vi "Get Channels from Line.vi"(11 "Line":T1={"channel"=refnum, "XNET Signal"="CANEventSignal1\nNIXNET_example.CAN_Cluster"}) -> (3 "Channels":refnum<class "TBM channel.lvclass">[](array[class]))   [LabVIEW 2014, in "J1939 configuration.lvclass"]
doc: "Returns an array of channels for a single line."
uses:
  J1939 configuration.lvclass
  <vilib>/NI/Tag Bus Module Framework/channel/TBM channel.lvclass
  Line.ctl
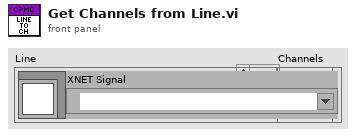
[diagram p1: front panel]
types:
  T1 = typedef "J1939 configuration.lvclass/Line.ctl" = cluster{"channel":refnum<class "TBM channel.lvclass">, "XNET Signal":refnum<k21>}
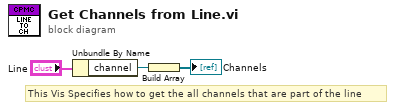
[diagram p0: block diagram]
diagram:
  # "This Vis Specifies how to get the all channels that are part of the line"
  n1 = Unbundle By Name("Line") -> ("channel"=w1:refnum<class "TBM channel.lvclass">)
  n2 = Build Array(w1) -> (→"Channels":refnum<class "TBM channel.lvclass">[])
